vi "ConfigureSignalTrackEnabled.vi"(8 "error in (no error)":errorcluster, 11 "Keysight44xx in":refnum<class "Keysight44xx.lvclass">) -> (0 "error out":errorcluster, 3 "Keysight44xx out":refnum<class "Keysight44xx.lvclass">)   [LabVIEW 2018, in "SpecAnPlugins.lvlib" / "Keysight44xx.lvclass"]
doc: "This VI turns signal-tracking on/off. When signal tracking is turned on, the spectrum analyzer centers the signal on which the active marker resides after each sweep. There are two prevalent methods of signal tracking in the industry. \n\n1. A search for the largest signal on screen is made, and the spectrum analyzer center frequency is tuned to this signal.\n\n2. The marker is placed on a signal (anywhere on screen) and when marker track is enabled, the frequency of the peak of the selected signal is used for tuning the spectrum analyzer. This does not need to be the largest signal on screen, and this method tracks the specified signal in the presence of a larger signal.\n\nThis VI implements the first method of signal tracking. This INVALIDATES the Frequency Start and Frequency Stop property values. \n\nNote: Signal track can only be enabled on one marker at a time. The driver shall check all other markers to see if this VI is already enabled on any marker other than the active and turn this off on the other marker before enabling this on the active marker."
uses:
  Keysight44xx.lvclass
  C:/Users/ico/Documents/Projects/NistPluggableModules/SpecAn/SpecAnPlugins/SpecAnBaseClass/SpecAnBase.lvclass
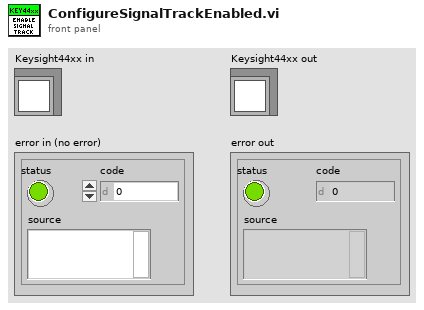
[diagram p1: front panel]
types:
  T1 = typedef "SpecAnPlugins.lvlib/SpecAnBase.lvclass/Acquisition.ctl" = cluster{"Handle":string, "Connected":bool, "Enabled":bool, "SweepModeContinuous":bool, "NumberOfSweeps":i32, "DetectorTypeAuto":bool, "DetectorType":i32, "VerticalScale":i32, "MaximumTime(seconds)":dbl}
  T2 = typedef "SpecAnPlugins.lvlib/SpecAnBase.lvclass/Markers.ctl" = cluster{"MarkerEnabled":bool, "MarkerThreshold":dbl, "PeakExcursion":dbl, "SignalTrackEnabled":bool, "MarkerPosition":dbl, "Instrument Setting (Frequency Center)":i32, "Marker search (Minimum)":i32, "ActiveMarker":string, "MarkerFrequencyCounter":bool, "FrequencyCounterResolution":dbl}
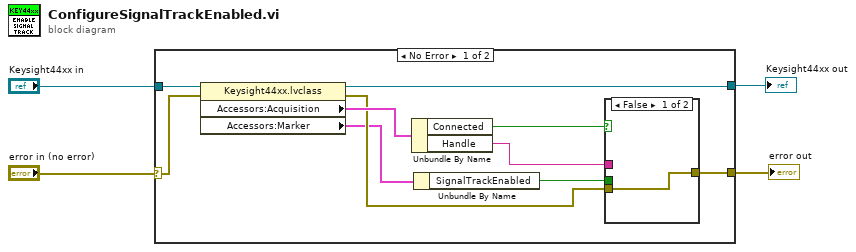
[diagram p0: block diagram]
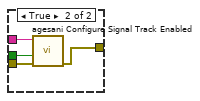
[diagram p2: hidden frame]
diagram:
  n1 = case shown="No Error" "error in (no error)" {
    selector: "error in (no error)" -> [w13 w20]
    tunnel: "Keysight44xx in" -> [w14 w21]
    tunnel: [w12 w21] -> w2
    tunnel: [w6 w20] -> w1
    frame No Error {
      n2 = property class="Keysight44xx.lvclass"(reference=w14, error in=w13) -> (reference out=w12:refnum<class "Keysight44xx.lvclass">, error out=w9:errorcluster, "Accessors:Acquisition"=w11:T1, "Accessors:Marker"=w8:T2)
      n3 = Unbundle By Name(w11) -> ("Connected"=w5:bool, "Handle"=w10:string)
      n4 = Unbundle By Name(w8) -> ("SignalTrackEnabled"=w7:bool)
      n5 = case shown="False" w5 {
        tunnel: w10 -> [_ w19]
        tunnel: w9 -> [w15 w18]
        tunnel: w7 -> [_ w17]
        tunnel: [w15 w16] -> w6
        frame False {
        }
        frame True {
          n6 = call <instrlib>:"agesani Configure Signal Track Enabled.vi"("error in (no error)"=w18, "signal track enabled (Off)"=w17, "instrument handle"=w19) -> ("error out"=w16:errorcluster)  [unwired: 7 in, 1 out]
        }
      }
    }
    frame Error {
    }
  }
  "error out" <- w1
  "Keysight44xx out" <- w2
